vi "ambient.vi"() -> ()   [LabVIEW 2011]
panel:
  in  "stop":bool
  in  "Start Measurement":bool
  in  "QUIT":bool
  in  "KILL":bool
  in  "PAUSE":bool
  in  "RESUME":bool
  out "standard error":string
  out "standard output":string
  # "Comandi di emergenza"
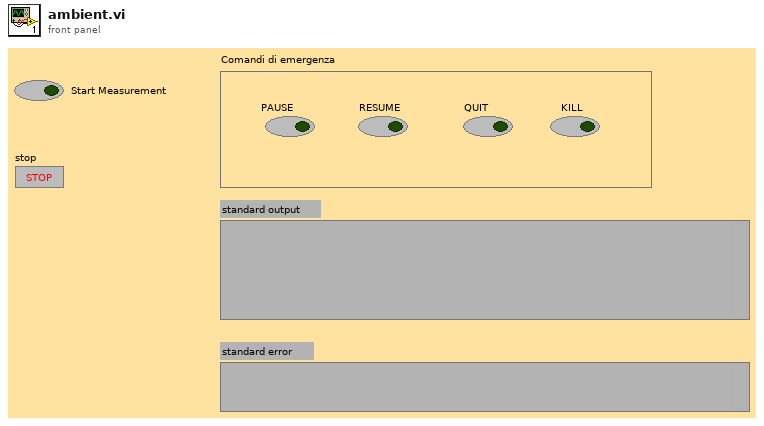
[diagram p1: front panel]
types:
  T1 = enum16{"open", "replace", "create", "open or create", "replace or create", "replace or create with confirmation"}
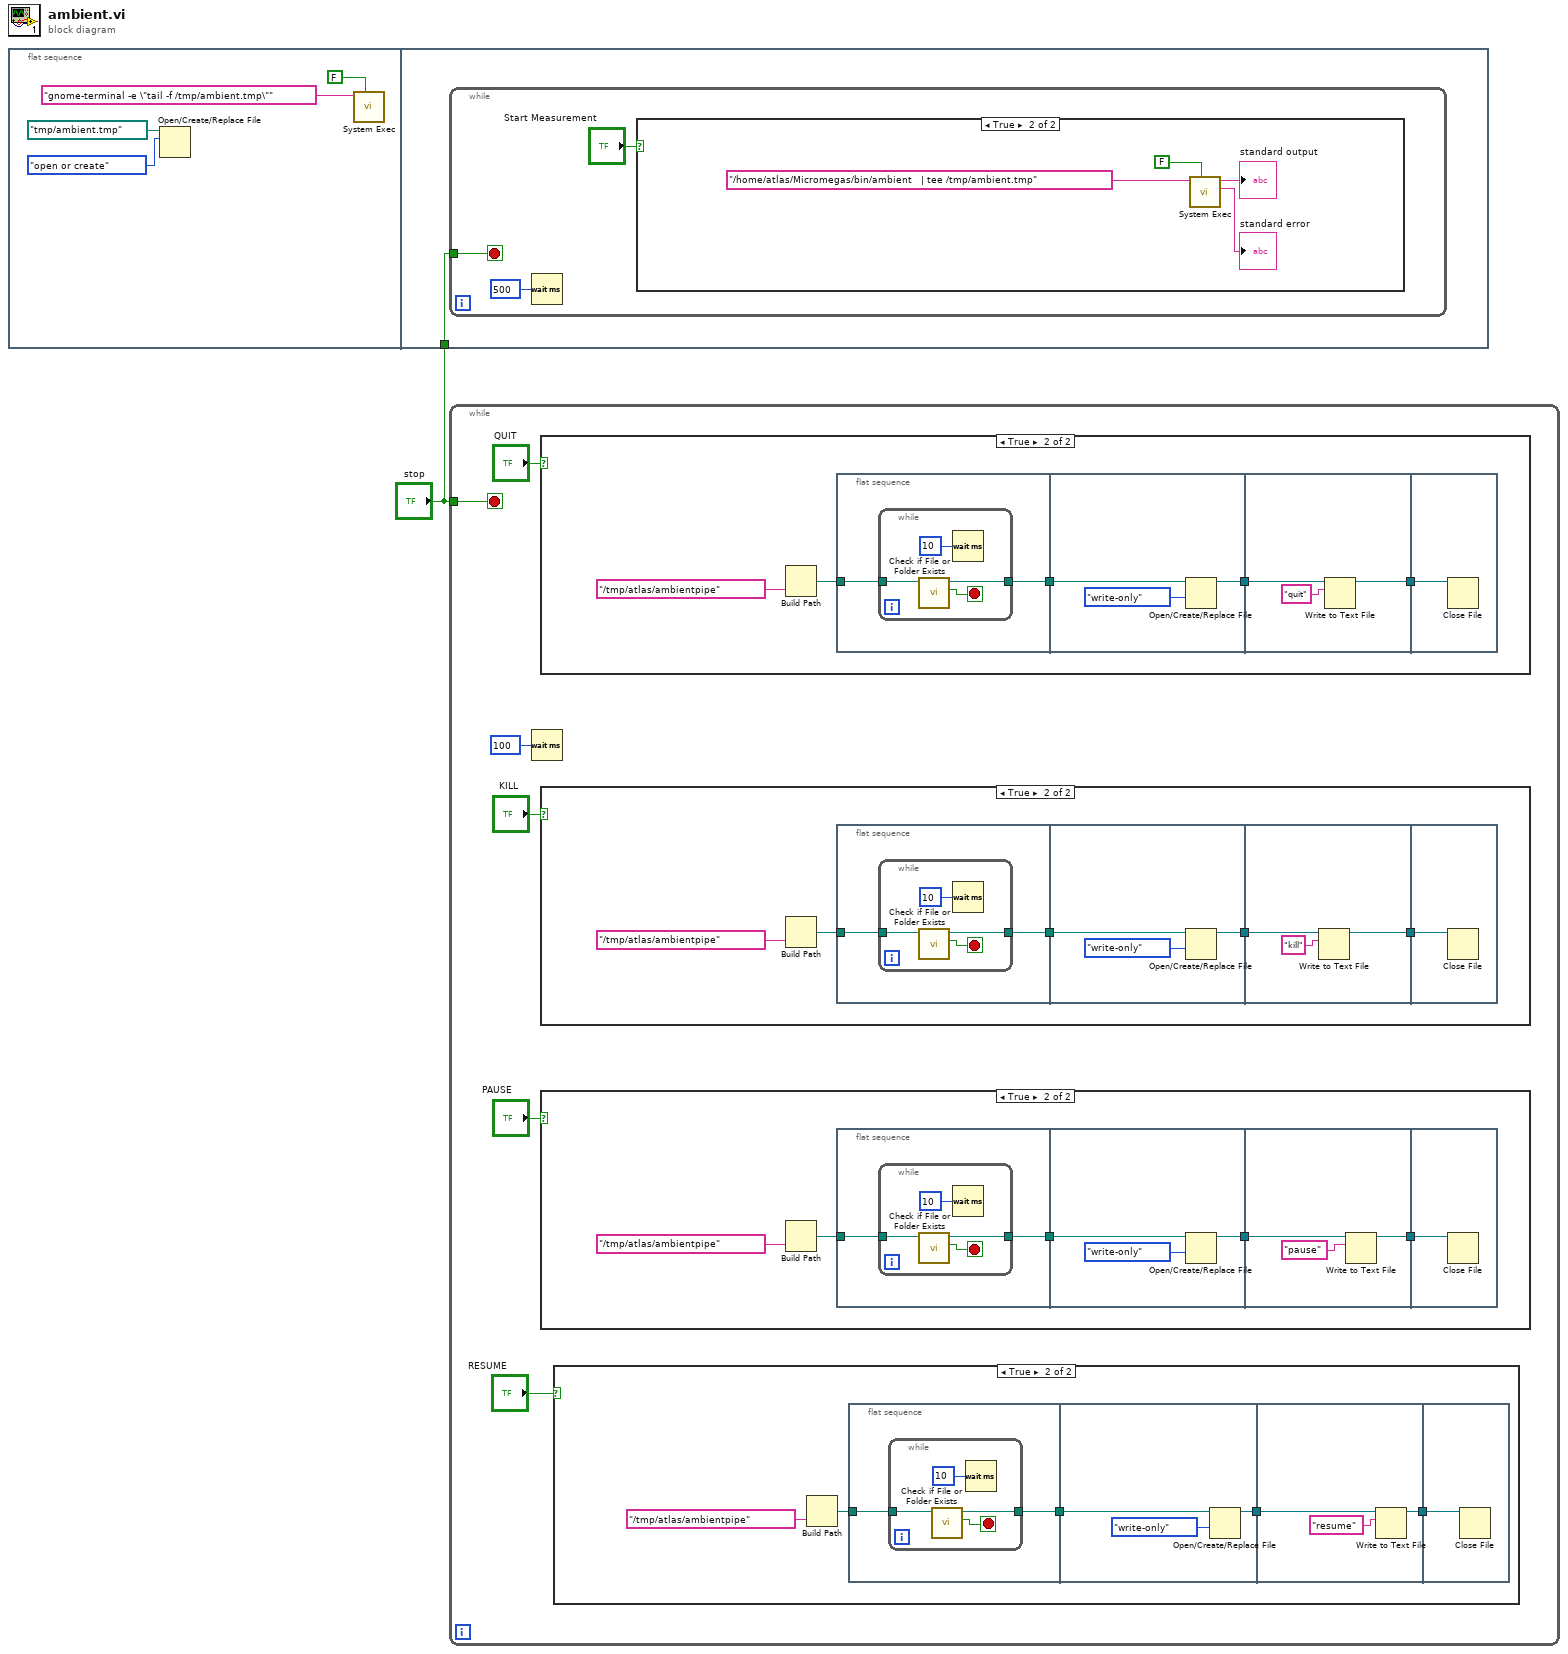
[diagram p0: block diagram]
diagram:
  n1 = flat-sequence {
    tunnel: "stop" -> [w6]
    frame #0 {
      n2 = Open/Create/Replace File(file path (use dialog)=path "/tmp/ambient.tmp", operation (0:open)=T1."open or create") -> ()  [unwired: 4 in, 3 out]
      n3 = call <vilib>:"System Exec.vi"("wait until completion? (T)"=FALSE, "command line"="gnome-terminal -e \"tail -f /tmp/ambient.tmp\"") -> ()  [unwired: 6 in, 4 out]
    }
    frame #1 {
      n4 = while {
        tunnel: w6 -> [w7]
        stop <- w7 stop-if-true
        n5 = Wait (ms)(milliseconds to wait=u32 500) -> ()  [unwired: 1 out]
        n6 = case shown="True" "Start Measurement" {
          frame False {
          }
          frame True {
            n7 = call <vilib>:"System Exec.vi"("wait until completion? (T)"=FALSE, "command line"="/home/atlas/Micromegas/bin/ambient   | tee /tmp/ambient.tmp") -> ("standard error"=→"standard error":string, "standard output"=→"standard output":string)  [unwired: 6 in, 2 out]
          }
        }
      }
    }
  }
  n8 = while {
    tunnel: "stop" -> [w14]
    stop <- w14 stop-if-true
    n9 = Wait (ms)(milliseconds to wait=100) -> ()  [unwired: 1 out]
    n10 = case shown="True" "QUIT" {
      frame False {
      }
      frame True {
        n11 = Build Path(name or relative path="/tmp/atlas/ambientpipe" ("string")) -> (appended path=w74:path)  [unwired: 1 in]
        n12 = flat-sequence {
          tunnel: [w80] -> w78
          tunnel: w74 -> [w79]
          tunnel: w78 -> [w87]
          tunnel: [w85] -> w77
          tunnel: w77 -> [w90]
          tunnel: [w89] -> w76
          tunnel: w76 -> [w91]
          frame #0 {
            n13 = while {
              tunnel: [w82] -> w80
              tunnel: w79 -> [w81]
              stop <- w83 stop-if-true
              n14 = call <vilib>:"Check if File or Folder Exists.vi"("path"=w81) -> ("file or folder exists?"=w83:bool, "dup path"=w82:path)  [unwired: 8 in, 1 out]
              n15 = Wait (ms)(milliseconds to wait=u32 10) -> ()  [unwired: 1 out]
            }
          }
          frame #1 {
            n16 = Open/Create/Replace File(file path (use dialog)=w87, access (0:read/write)=enum16{"read/write", "read-only", "write-only"}."write-only") -> (refnum out=w85:refnum<file>)  [unwired: 4 in, 2 out]
          }
          frame #2 {
            n17 = Write to Text File(file (use dialog)=w90, text="quit") -> (refnum out=w89:refnum<file>)  [unwired: 2 in, 2 out]
          }
          frame #3 {
            n18 = Close File(refnum=w91) -> ()  [unwired: 1 in, 2 out]
          }
        }
      }
    }
    n19 = case shown="True" "KILL" {
      frame False {
      }
      frame True {
        n20 = Build Path(name or relative path="/tmp/atlas/ambientpipe" ("string")) -> (appended path=w38:path)  [unwired: 1 in]
        n21 = flat-sequence {
          tunnel: [w44] -> w42
          tunnel: w38 -> [w43]
          tunnel: w42 -> [w51]
          tunnel: [w49] -> w41
          tunnel: w41 -> [w54]
          tunnel: [w53] -> w40
          tunnel: w40 -> [w55]
          frame #0 {
            n22 = while {
              tunnel: [w46] -> w44
              tunnel: w43 -> [w45]
              stop <- w47 stop-if-true
              n23 = call <vilib>:"Check if File or Folder Exists.vi"("path"=w45) -> ("file or folder exists?"=w47:bool, "dup path"=w46:path)  [unwired: 8 in, 1 out]
              n24 = Wait (ms)(milliseconds to wait=u32 10) -> ()  [unwired: 1 out]
            }
          }
          frame #1 {
            n25 = Open/Create/Replace File(file path (use dialog)=w51, access (0:read/write)=enum16{"read/write", "read-only", "write-only"}."write-only") -> (refnum out=w49:refnum<file>)  [unwired: 4 in, 2 out]
          }
          frame #2 {
            n26 = Write to Text File(file (use dialog)=w54, text="kill") -> (refnum out=w53:refnum<file>)  [unwired: 2 in, 2 out]
          }
          frame #3 {
            n27 = Close File(refnum=w55) -> ()  [unwired: 1 in, 2 out]
          }
        }
      }
    }
    n28 = case shown="True" "PAUSE" {
      frame False {
      }
      frame True {
        n29 = Build Path(name or relative path="/tmp/atlas/ambientpipe" ("string")) -> (appended path=w20:path)  [unwired: 1 in]
        n30 = flat-sequence {
          tunnel: [w26] -> w24
          tunnel: w20 -> [w25]
          tunnel: w24 -> [w33]
          tunnel: [w31] -> w23
          tunnel: w23 -> [w36]
          tunnel: [w35] -> w22
          tunnel: w22 -> [w37]
          frame #0 {
            n31 = while {
              tunnel: [w28] -> w26
              tunnel: w25 -> [w27]
              stop <- w29 stop-if-true
              n32 = call <vilib>:"Check if File or Folder Exists.vi"("path"=w27) -> ("file or folder exists?"=w29:bool, "dup path"=w28:path)  [unwired: 8 in, 1 out]
              n33 = Wait (ms)(milliseconds to wait=u32 10) -> ()  [unwired: 1 out]
            }
          }
          frame #1 {
            n34 = Open/Create/Replace File(file path (use dialog)=w33, access (0:read/write)=enum16{"read/write", "read-only", "write-only"}."write-only") -> (refnum out=w31:refnum<file>)  [unwired: 4 in, 2 out]
          }
          frame #2 {
            n35 = Write to Text File(file (use dialog)=w36, text="pause") -> (refnum out=w35:refnum<file>)  [unwired: 2 in, 2 out]
          }
          frame #3 {
            n36 = Close File(refnum=w37) -> ()  [unwired: 1 in, 2 out]
          }
        }
      }
    }
    n37 = case shown="True" "RESUME" {
      frame False {
      }
      frame True {
        n38 = Build Path(name or relative path="/tmp/atlas/ambientpipe" ("string")) -> (appended path=w56:path)  [unwired: 1 in]
        n39 = flat-sequence {
          tunnel: [w62] -> w60
          tunnel: w56 -> [w61]
          tunnel: w60 -> [w69]
          tunnel: [w67] -> w59
          tunnel: w59 -> [w72]
          tunnel: [w71] -> w58
          tunnel: w58 -> [w73]
          frame #0 {
            n40 = while {
              tunnel: [w64] -> w62
              tunnel: w61 -> [w63]
              stop <- w65 stop-if-true
              n41 = call <vilib>:"Check if File or Folder Exists.vi"("path"=w63) -> ("file or folder exists?"=w65:bool, "dup path"=w64:path)  [unwired: 8 in, 1 out]
              n42 = Wait (ms)(milliseconds to wait=u32 10) -> ()  [unwired: 1 out]
            }
          }
          frame #1 {
            n43 = Open/Create/Replace File(file path (use dialog)=w69, access (0:read/write)=enum16{"read/write", "read-only", "write-only"}."write-only") -> (refnum out=w67:refnum<file>)  [unwired: 4 in, 2 out]
          }
          frame #2 {
            n44 = Write to Text File(file (use dialog)=w72, text="resume") -> (refnum out=w71:refnum<file>)  [unwired: 2 in, 2 out]
          }
          frame #3 {
            n45 = Close File(refnum=w73) -> ()  [unwired: 1 in, 2 out]
          }
        }
      }
    }
  }
